vi "Motion Profle To Array.vi"(8 "Encoder Units":dbl, 9 "Wheel Diameter (M)":dbl, 11 "path":dbl[][](array[numeric])) -> (3 "Motion Profile Trajectory Point Array":T1[](array[typedef]))   [LabVIEW 2020]
uses:
  <vilib>/Rock Robotics/WPI/ThirdParty/Phoenix-LabVIEW/Motor Controller/Controls/CTRE_Phoenix_MotorControl_MotionProfileTrajectoryPoint.ctl
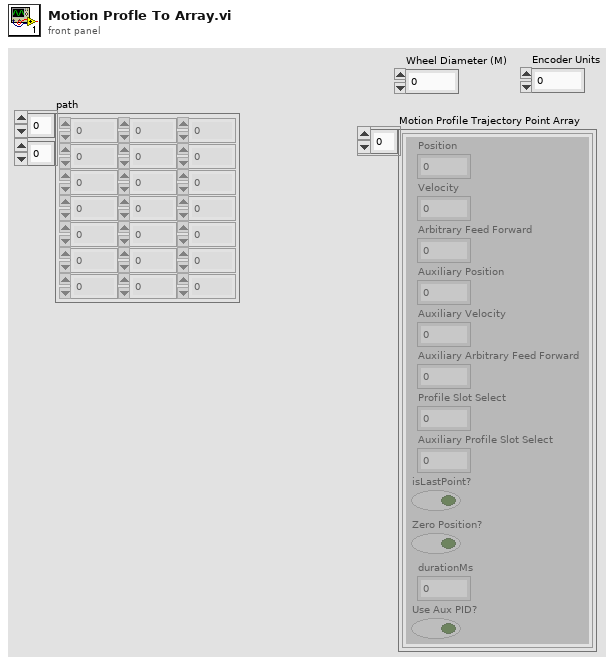
[diagram p1: front panel]
types:
  T1 = typedef "CTRE_Phoenix_MotorControl_MotionProfileTrajectoryPoint.ctl" = cluster{"Position":dbl, "Velocity":dbl, "Arbitrary Feed Forward":dbl, "Auxiliary Position":dbl, "Auxiliary Velocity":dbl, "Auxiliary Arbitrary Feed Forward":dbl, "Profile Slot Select":i32, "Auxiliary Profile Slot Select":i32, "isLastPoint?":bool, "Zero Position?":bool, "durationMs":u32, "Use Aux PID?":bool}
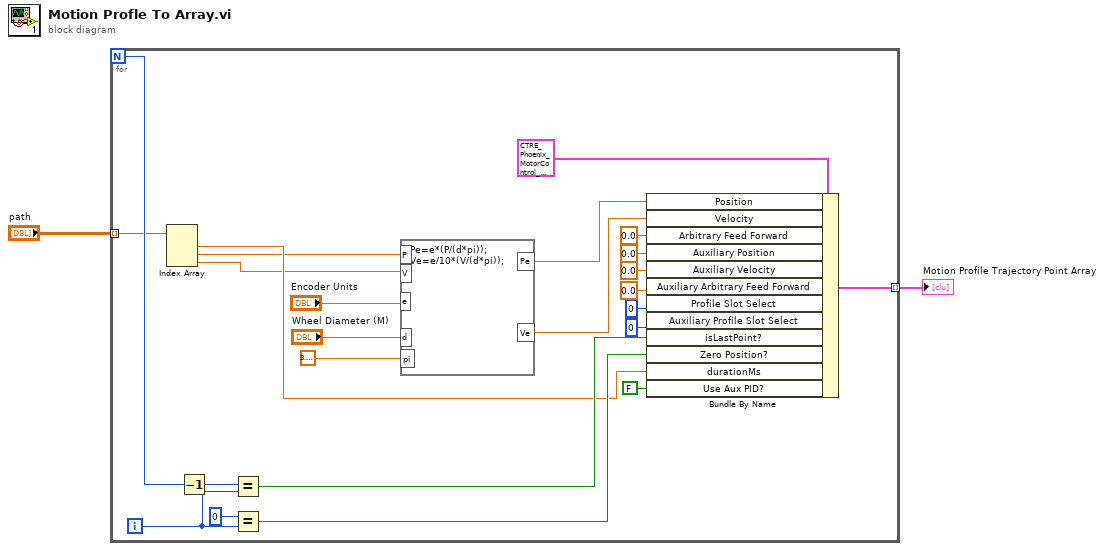
[diagram p0: block diagram]
diagram:
  n1 = for {
    N -> [w12]
    tunnel: [w23] -> w2 mode=indexing
    tunnel: "path" -> [w6] mode=indexing
    i -> [w9]
    n2 = Index Array(array=w6) -> (element #1=w5:dbl, element #2=w4:dbl, element #3=w3:dbl)  [unwired: 3 in]
    n3 = Decrement(x=w12) -> (x-1=w10:i32)
    n4 = Equal?(x=w10, y=w9) -> (x = y?=w8:bool)
    n5 = Equal?(x=0, y=w9) -> (x = y?=w13:bool)
    n6 = formula code="Pe=e*(P/(d*pi));\nVe=e/10*(V/(d*pi));"("P"=w4, "d"="Wheel Diameter (M)", "pi"=3.141592653589793, "V"=w3, "e"="Encoder Units") -> ("Pe"=w21:dbl, "Ve"=w20:dbl)
    n7 = Bundle By Name(cluster=T1 {"Position"=0.0, "Velocity"=0.0, "Arbitrary Feed Forward"=0.0, "Auxiliary Position"=0.0, "Auxiliary Velocity"=0.0, "Auxiliary Arbitrary Feed Forward"=0.0, "Profile Slot Select"=0, "Auxiliary Profile Slot Select"=0, "isLastPoint?"=FALSE, "Zero Position?"=FALSE, "durationMs"=0, "Use Aux PID?"=FALSE} ("Trajectory Point"), "Position"=w21, "Velocity"=w20, "Arbitrary Feed Forward"=0.0, "Auxiliary Position"=0.0, "Auxiliary Velocity"=0.0, "Auxiliary Arbitrary Feed Forward"=0.0, "Profile Slot Select"=0, "Auxiliary Profile Slot Select"=0, "isLastPoint?"=w8, "Zero Position?"=w13, "durationMs"=w5, "Use Aux PID?"=FALSE) -> (w23:T1)
  }
  "Motion Profile Trajectory Point Array" <- w2
